vi "SD Read Numeric Array.vi"(8 "error in":errorcluster, 10 "Table Prefix":string="SmartDashboard", 11 "Name":string="Numeric Array") -> (0 "error out":errorcluster, 2 "Table Prefix out":string, 3 "Numeric Array":dbl[](array[numeric]))   [LabVIEW 2017]
doc: "Return the double precision numeric array data stored in the SmartDashboard entry -- /prefix/name. Return an error if not present or not a numeric array."
uses:
  <vilib>/Rock Robotics/Network Tables/Field Type.ctl
  <vilib>/Rock Robotics/Network Tables/Field Data Manager.vi
  <vilib>/Rock Robotics/Network Tables/Table Manager.vi
  <vilib>/Rock Robotics/Network Tables/Prepare Table Name.vi
  <vilib>/Rock Robotics/Network Tables/Usage Statistics.vi
  <vilib>/Rock Robotics/Network Tables/NT Globals.vi
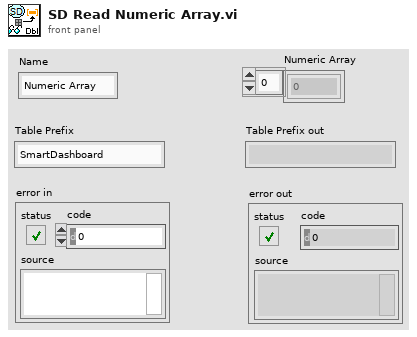
[diagram p1: front panel]
types:
  T1 = typedef "Field Type.ctl" = enum8{"Invalid", "Bool", "Numeric", "String", "Raw", "Boolean Array", "Numeric Array", "String Array", "RPC"}
  T2 = typedef "Field Data.ctl" = cluster{"Dbl":dbl, "String":string, "Type":T1, "Boolean":bool, "Sequence #":T3, "Flags":u8}
  T3 = typedef "Sequence.ctl" = u16
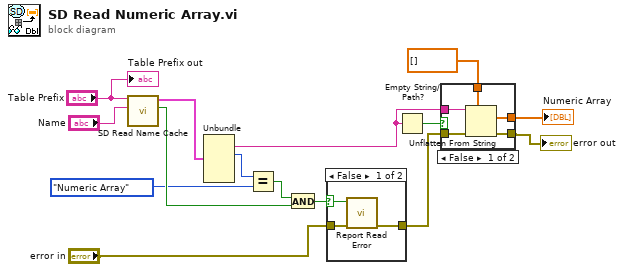
[diagram p0: block diagram]
diagram:
  n1 = call <vilib>:"SD Read Name Cache.vi"("Name"="Name", "Table Prefix"="Table Prefix") -> ("Success"=w15:bool, "Field Value Out"=w14:T2)  [unwired: 8 in]
  n2 = Unbundle(w14) -> ("String"=w3:string, "Type"=w11:T1)  [unwired: 4 out]
  n3 = Equal?(x=w11, y=Field_Type."Numeric Array" ("Type")) -> (x = y?=w13:bool)
  n4 = And(x=w13, y=w15) -> (x .and. y?=w10:bool)
  n5 = case shown="False" w10 {
    selector: w10 -> [w16 _]
    tunnel: [w18 w19] -> w4
    tunnel: "error in" -> [w17 w19]
    frame False {
      n6 = call <vilib>:"Report Read Error.vi"("error in (no error)"=w17, "Success"=w16) -> ("error out"=w18:errorcluster)  [unwired: 9 in]
    }
    frame True {
    }
  }
  n7 = Empty String/Path?(string/path=w3) -> (empty?=w6:bool)
  n8 = case shown="False" w6 {
    tunnel: w3 -> [w24 _]
    tunnel: dbl[] [] ("Boolean Array") -> [w23 w26]
    tunnel: [w22 w26] -> w2
    tunnel: [w21 w25] -> w1
    tunnel: w4 -> [w20 w25]
    frame False {
      n9 = Unflatten From String(type=w23, binary string=w24, error in (no error)=w20) -> (value=w22:dbl[], error out=w21:errorcluster)  [unwired: 2 in, 1 out]
    }
    frame True {
    }
  }
  "Numeric Array" <- w2
  "error out" <- w1
  "Table Prefix out" <- "Table Prefix"
